vi "BotSpeakSerial_Init1.vi"(3 "StartupWait":i32, 4 "Com Protocol":string, 5 "Address":string) -> (0 "error out":errorcluster)   [LabVIEW 2012]
uses:
  <userlib>/botspeak/VIs/SubVIs/BotSpeak_Globals.vi
  <vilib>/Instr/_visa.llb/VISA Configure Serial Port (Instr).vi
panel:
  out "error out 2":errorcluster
  out "VISA resource name out":refnum<visa-resource-name>
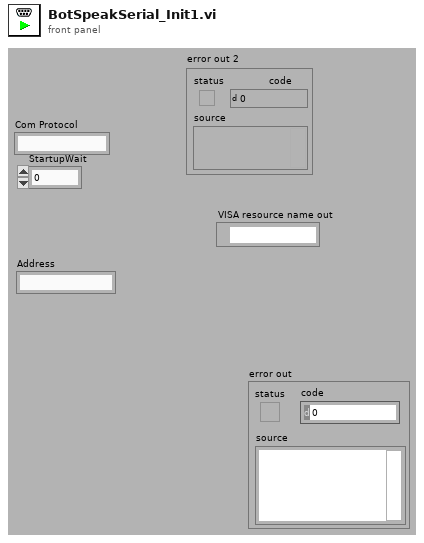
[diagram p1: front panel]
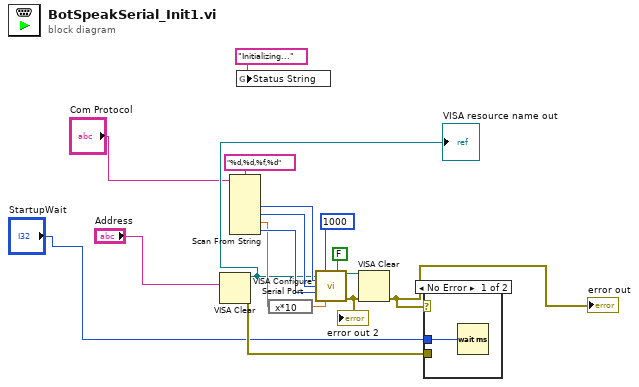
[diagram p0: block diagram]
diagram:
  n1 = VISA Clear(VISA resource name="Address") -> (VISA resource name out=w7:refnum<visa-resource-name>, error out=w5:errorcluster)  [unwired: 1 in]
  "VISA resource name out" <- w7
  n2 = Scan From String(format string="%d,%d,%f,%d", input string="Com Protocol") -> (output 1=w10:i32, output 2=w11:i32, output 3=w12:dbl, output 4=w13:i32)  [unwired: 6 in, 3 out]
  n3 = global write "BotSpeak_Globals.vi" "Status String"("Initializing..." ("Status String")) -> ()
  n4 = expression code="x*10"(w12) -> (w14:dbl)
  n5 = call-poly "VISA Configure Serial Port"("VISA resource name"=w7, "timeout (10sec)"=u32 1000, "Enable Termination\nChar (T)"=FALSE ("Enable Termination\nChar (T)"), "baud rate (9600)"=w10, "data bits (8)"=w11, "parity (0:none)"=w13, "stop bits (10: 1 bit)"=w14) -> ("VISA resource name out"=w4:refnum<visa-resource-name>, "error out"=w3:errorcluster)  [unwired: 7 in]
  "error out 2" <- w3
  n6 = VISA Clear(VISA resource name=w4, error in (no error)=w3) -> (error out=w15:errorcluster)  [unwired: 1 out]
  "error out" <- w15
  n7 = case shown="No Error" w15 {
    tunnel: "StartupWait" -> [w18 _]
    tunnel: w5 -> [_ _]
    frame No Error {
      n8 = Wait (ms)(milliseconds to wait=w18) -> ()  [unwired: 1 out]
    }
    frame Error {
    }
  }
